vi "LabView Code.vi"() -> ()   [LabVIEW 2021]
panel:
  in  "Voltage 0":bool=TRUE caption="Enable"
  out "Waveform Graph":dynamicdata(graph)
  out "Save Data":bool=TRUE caption="Enable"
  out "Seconds":dbl
  in  "rate":dbl=100000.0
  in  "number of samples":i32=300000
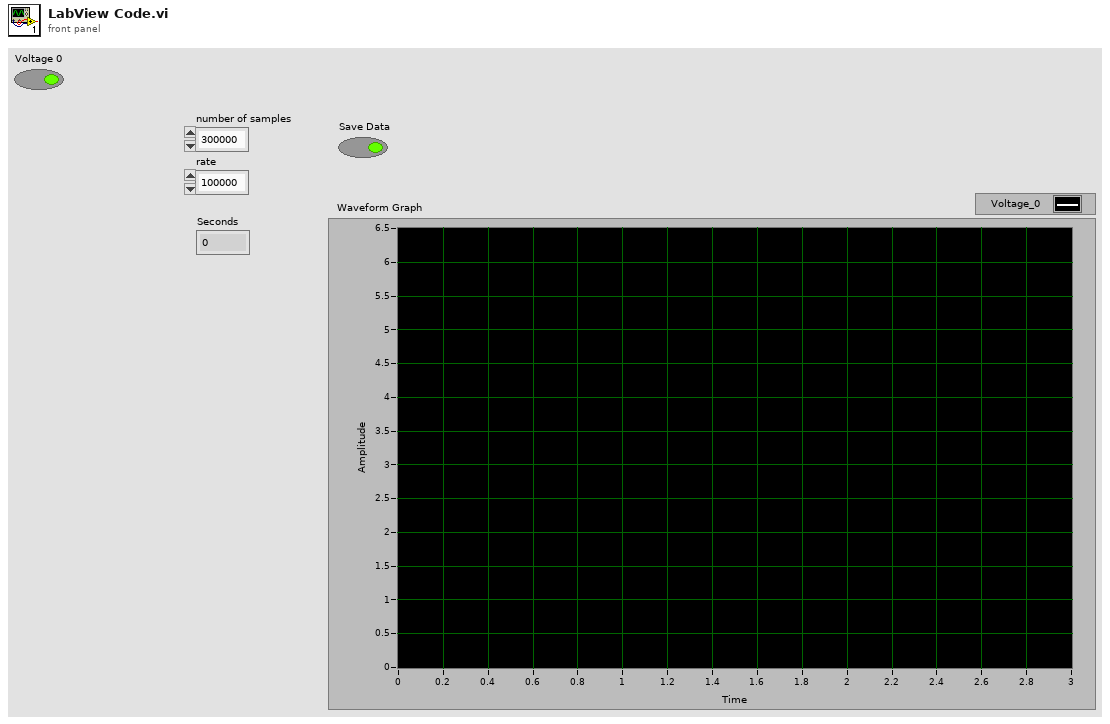
[diagram p1: front panel]
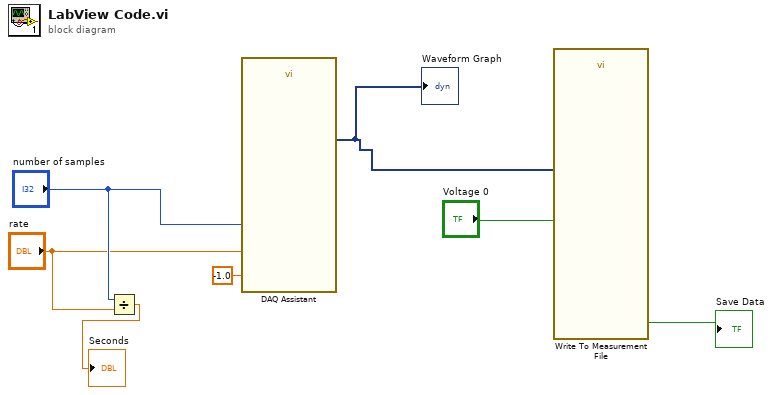
[diagram p0: block diagram]
diagram:
  n1 = Divide(x="number of samples", y="rate") -> (x/y=→"Seconds":dbl)
  n2 = call "DAQ Assistant"("rate"="rate", "number of samples"="number of samples", "timeout (s)"=-1.0) -> ("data"=w2:dynamicdata)  [unwired: 14 in, 2 out]
  "Waveform Graph" <- w2
  n3 = call "Write To Measurement File"("Signals"=w2, "Enable"="Voltage 0") -> ("Saving Data"=→"Save Data":bool)  [unwired: 15 in, 2 out]
